vi "Digital Serial Gen Cfg Popup.vi"(8 "error in (no error)":errorcluster, 11 "config file in":path caption="Configuration File") -> (0 "error out":errorcluster, 2 "digital audio protocol settings":T1={"number of channels"=0, "data justification"=enum."Left Justified", "endianness"=enum."LSB First", "channel length"=0, "bit depth"=0, "frame clock rate"=0.0, "bit clock edge sync"=enum."Falling", "master clock rate"=0.0, "Logic Level"=enum."1.2 V", "frame sync edge for channel 0"=enum."Rising", "Channel 0 Offset"=0}, 3 "config file out":path caption="Configuration File")   [LabVIEW 2021, in "Audio Popup UI.lvlib"]
uses:
  Audio Popup UI.lvlib
  controls/digital serial gen settings.ctl
  <vilib>/PDM Acquisition Toolkit/shared/controls/PCM Data Justification.ctl
  <vilib>/PDM Acquisition Toolkit/shared/controls/PCM Bit Endianness.ctl
  <vilib>/PDM Acquisition Toolkit/shared/controls/Digital Edge.ctl
  <vilib>/PDM Acquisition Toolkit/host/Classes/Session/Controls/Logic Levels.ctl
  <vilib>/Utility/miscctls.llb/LVPointTypeDef.ctl
  <vilib>/PDM Acquisition Toolkit/shared/PDM Shared.lvlib
  <vilib>/PDM Acquisition Toolkit/host/Classes/Session/DecoderSession.lvclass
  digital serial gen settings/digital audio protocol controls.lvlib
panel:
  in  "channel 0 offset":u32=1
  in  "Save":bool
  in  "logic level":enum32{"3.3 V", "1.8 V", "1.2 V"}(ring) caption="Logic level"
  in  "master clock rate":dbl=12288000.0 caption="Master clock rate" format="%#_6pHz"
  out "Bit clock rate":dbl=3072000.0 format="%#_6pHz"
  in  "number of channels":u32=2 caption="Number of channels"
  in  "TDM":bool
  in  "RJ":bool
  in  "LJ":bool
  in  "I2S":bool
  in  "bit clock edge sync":enum32{"Rising", "Falling"}(ring)=enum."Falling" caption="Bit clock edge sync"
  in  "frame clock rate":dbl=48000.0 caption="Frame clock rate" format="%#_6pHz"
  in  "data justification":enum32{"Left Justified", "Right Justified"}(ring) caption="Data justification"
  in  "endianness":enum32{"MSB First", "LSB First"}(ring) caption="Endianness"
  in  "bit depth":u32=24 caption="Bit depth"
  in  "channel length":u32=32 caption="Channel length"
  in  "frame sync edge for channel 0":enum32{"Rising", "Falling"}(ring)=enum."Falling" caption="Frame sync edge for Channel 0"
  # "Audio Protocol"
  # "Clock Settings"
  # "Signal Level"
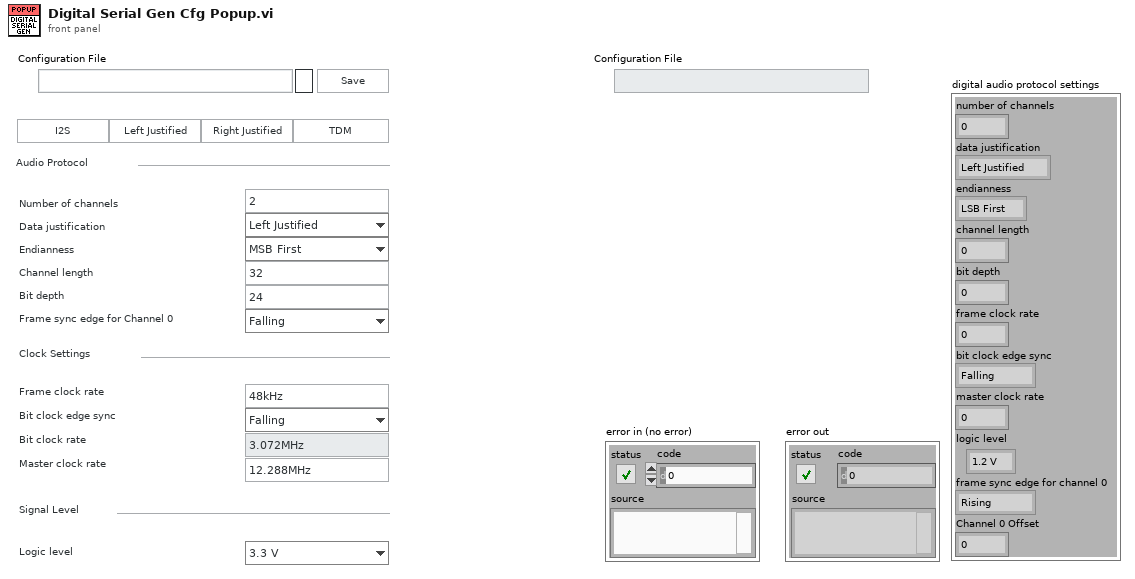
[diagram p1: front panel]
types:
  T1 = typedef "digital serial gen settings.ctl" = cluster{"number of channels":u32, "data justification":T2, "endianness":T3, "channel length":u32, "bit depth":u32, "frame clock rate":dbl, "bit clock edge sync":T4, "master clock rate":dbl, "Logic Level":T5, "frame sync edge for channel 0":T4, "Channel 0 Offset":u32}
  T2 = typedef "PDM Shared.lvlib/PCM Data Justification.ctl" = enum16{"Left Justified", "Right Justified"}
  T3 = typedef "PDM Shared.lvlib/PCM Bit Endianness.ctl" = enum16{"MSB First", "LSB First"}
  T4 = typedef "PDM Shared.lvlib/Digital Edge.ctl" = enum8{"Rising", "Falling"}
  T5 = typedef "PDM Acquisition Class Library.lvlib/DecoderSession.lvclass/Logic Levels.ctl" = enum16{"3.3 V", "1.8 V", "1.2 V"}
  T6 = typedef "LVPointTypeDef.ctl" = cluster{"Horizontal":i16, "Vertical":i16}
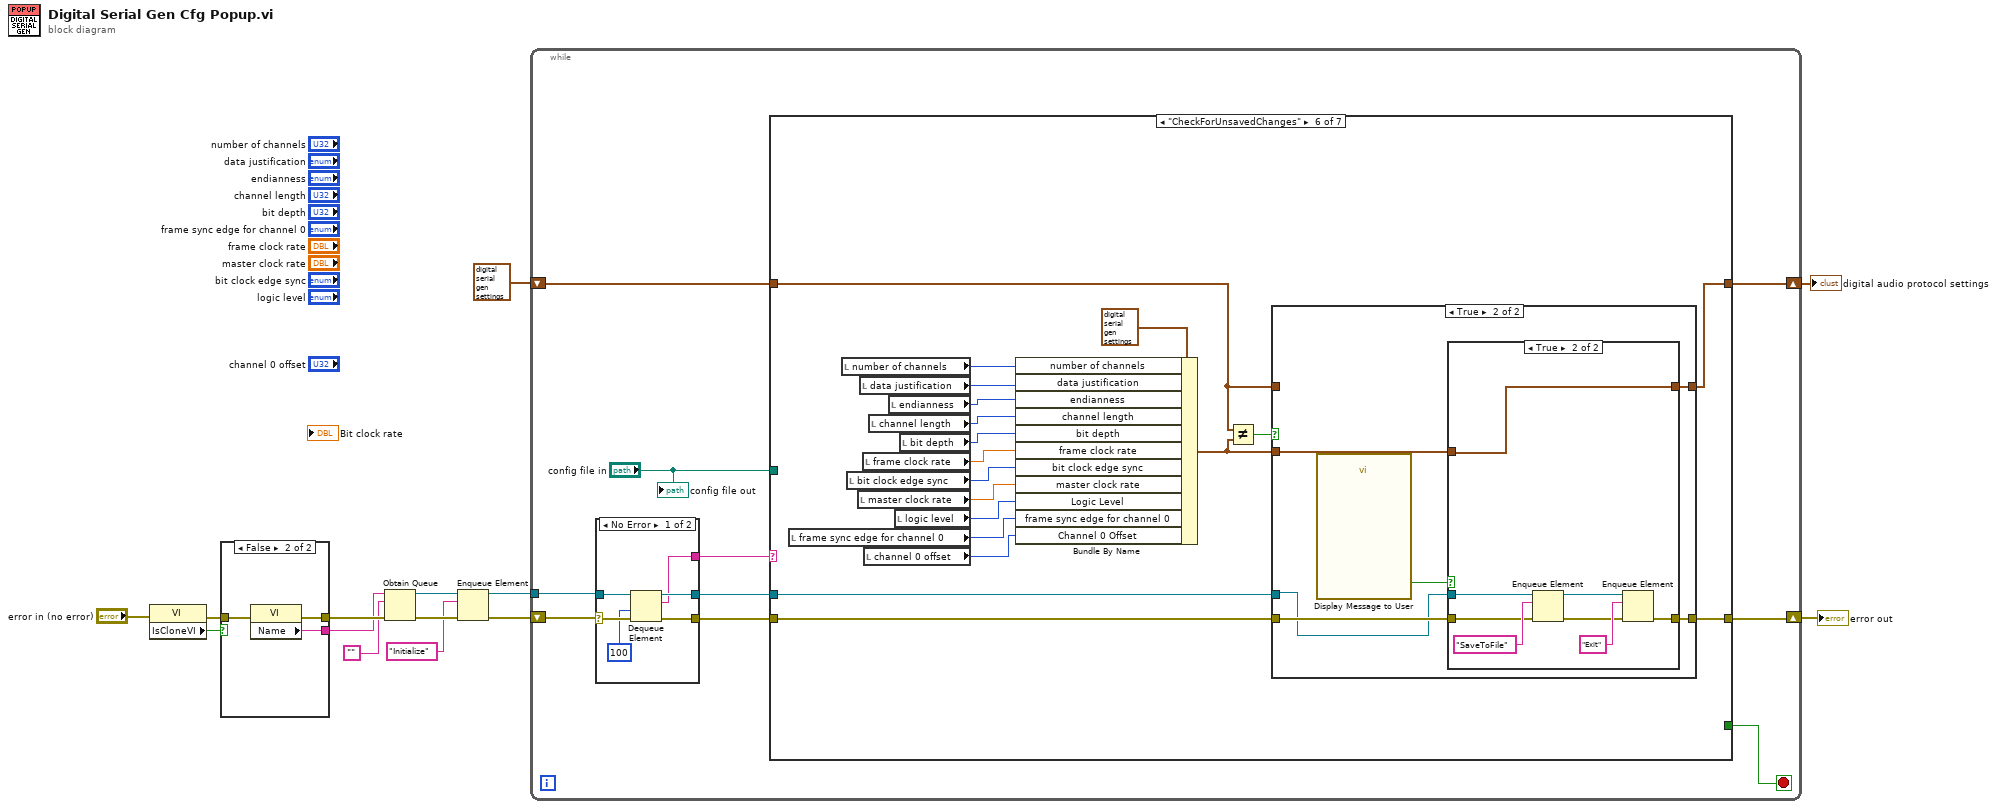
[diagram p0: block diagram]
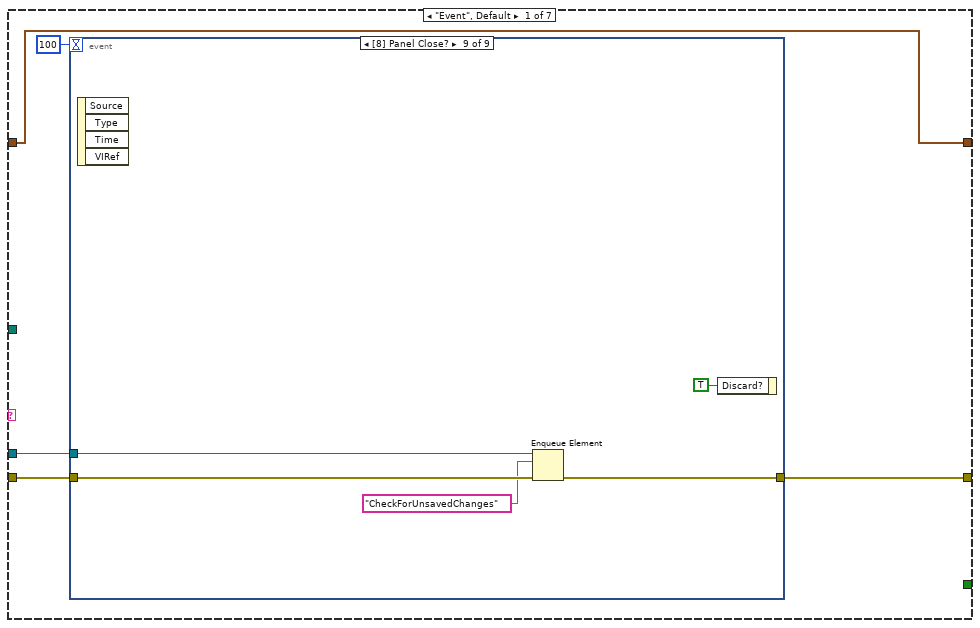
[diagram p2: hidden frame]
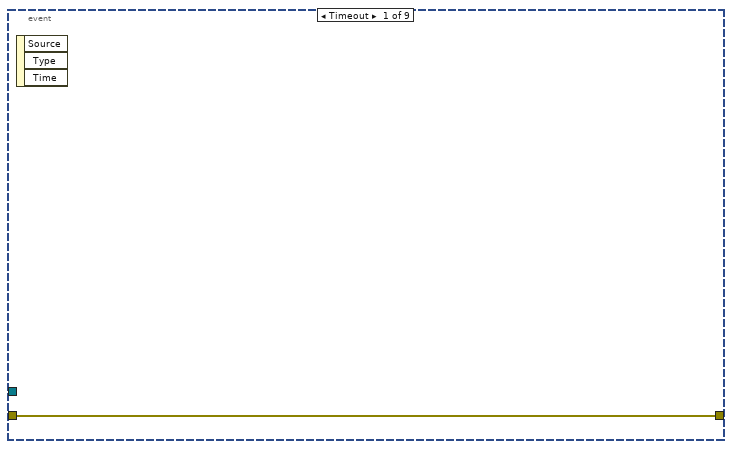
[diagram p3: hidden frame]
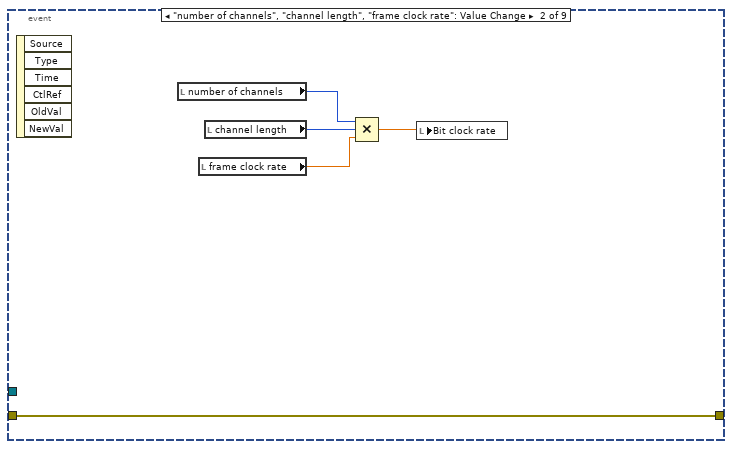
[diagram p4: hidden frame]
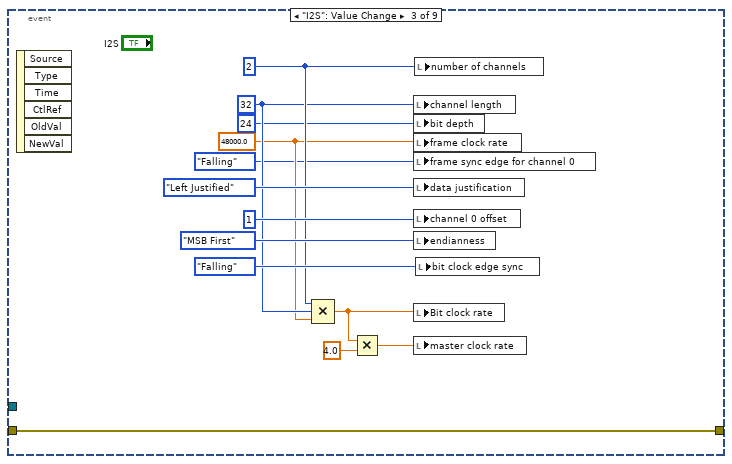
[diagram p5: hidden frame]
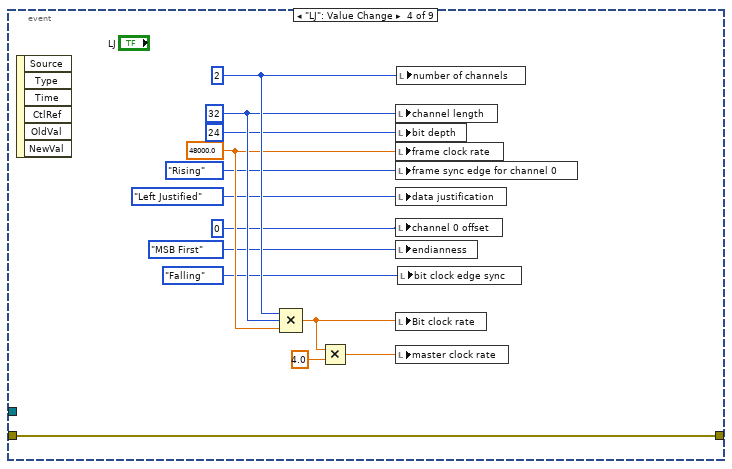
[diagram p6: hidden frame]
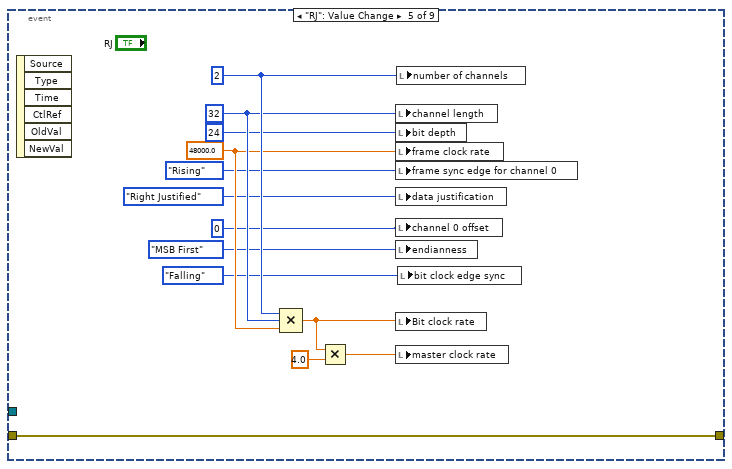
[diagram p7: hidden frame]
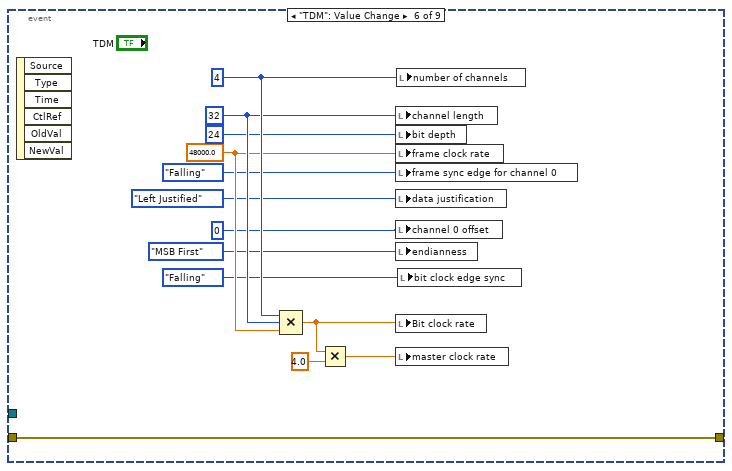
[diagram p8: hidden frame]
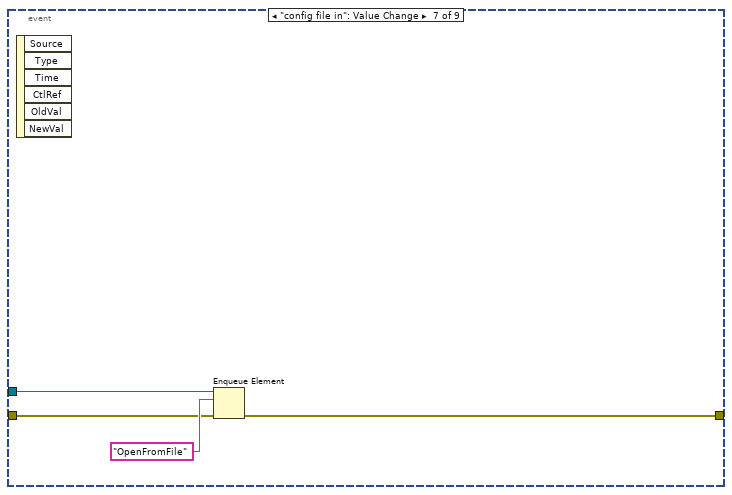
[diagram p9: hidden frame]
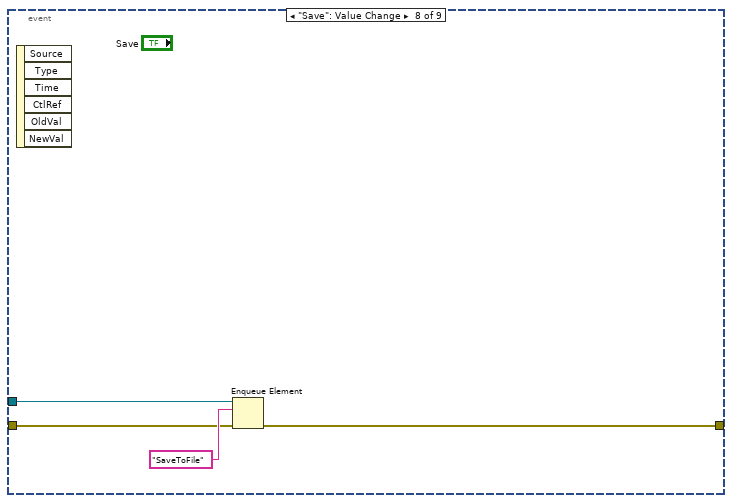
[diagram p10: hidden frame]
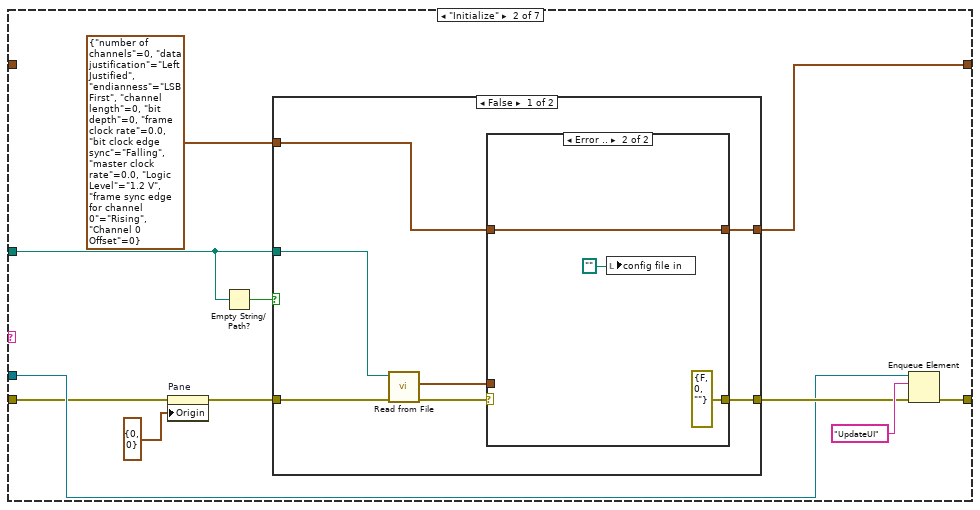
[diagram p11: hidden frame]
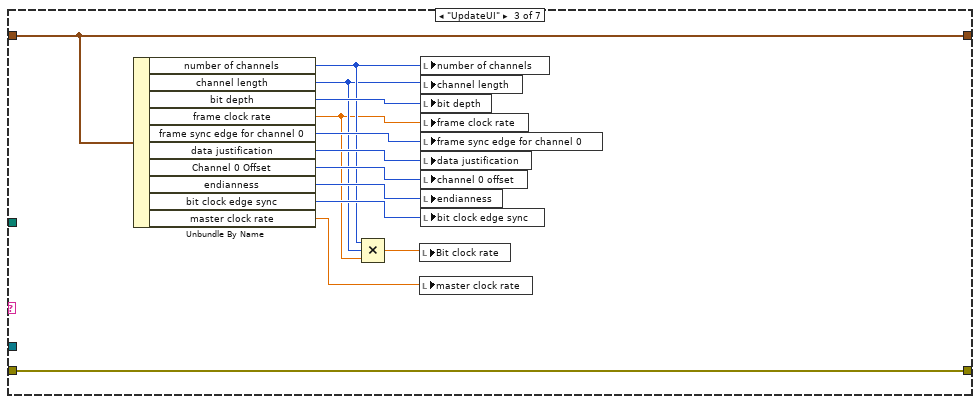
[diagram p14: hidden frame]
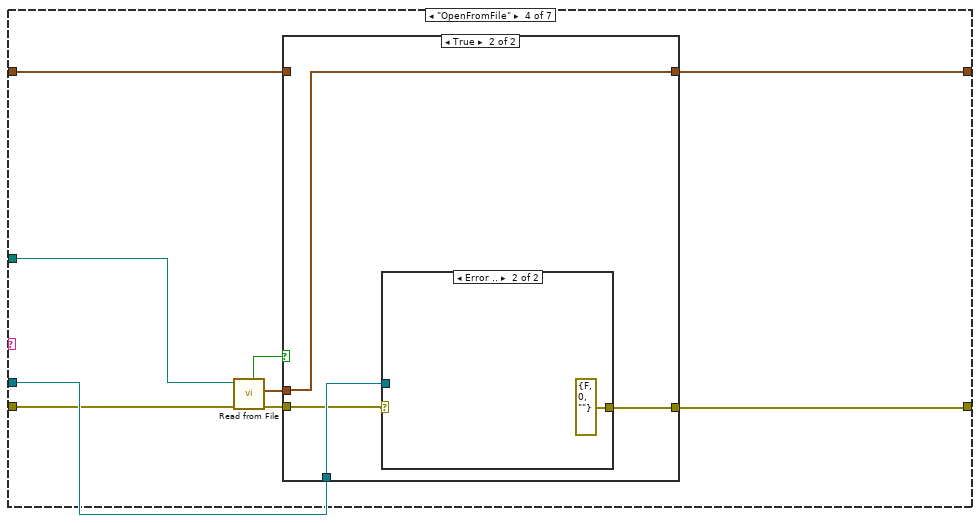
[diagram p15: hidden frame]
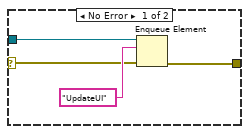
[diagram p17: hidden frame]
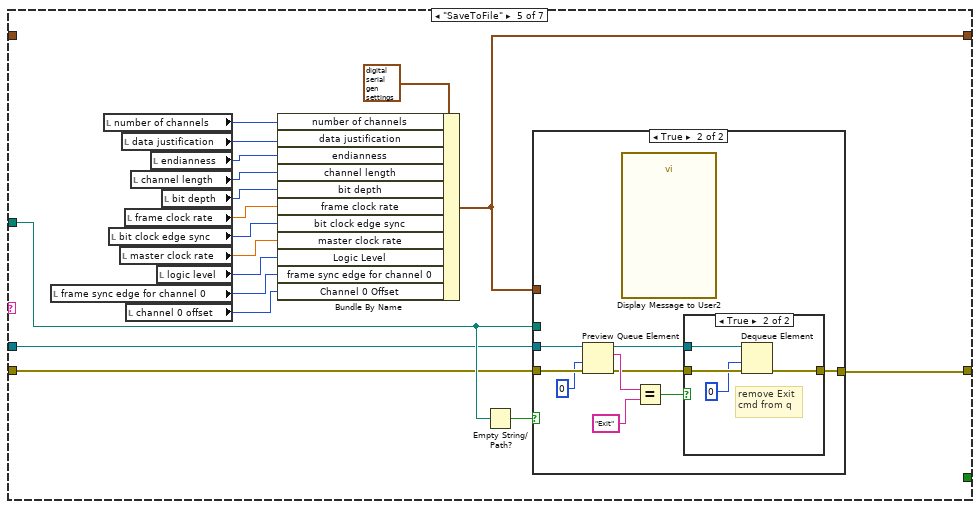
[diagram p18: hidden frame]
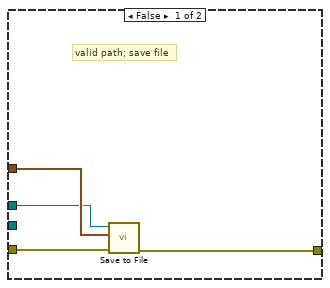
[diagram p19: hidden frame]
diagram:
  n1 = property class="VI"(error in="error in (no error)") -> (error out=w7:errorcluster, "IsCloneVI"=w8:bool)  [unwired: 1 in, 1 out]
  n2 = case shown="False" w8 {
    tunnel: [w17 w20] -> w14
    tunnel: [w16 w19] -> w13
    tunnel: w7 -> [w15 w18]
    frame True {
      n3 = property class="VI"(error in=w15) -> (error out=w17:errorcluster, "Clone Name"=w16:string)  [unwired: 1 in, 1 out]
    }
    frame False {
      n4 = property class="VI"(error in=w18) -> (error out=w20:errorcluster, "Name"=w19:string)  [unwired: 1 in, 1 out]
    }
  }
  n5 = Obtain Queue(name (unnamed)=w13, element data type="", error in (no error)=w14) -> (queue out=w11:refnum<queue>, error out=w12:errorcluster)  [unwired: 2 in, 1 out]
  n6 = Enqueue Element(queue=w11, element="Initialize", error in (no error)=w12) -> (queue out=w5:refnum<queue>, error out=w6:errorcluster)  [unwired: 1 in, 1 out]
  n7 = while {
    tunnel: w5 -> [w29]
    shift-right: [w25] -> w3
    shift-left: w6 -> [w30]
    shift-right: [w22] -> w1
    shift-left: T1 {"number of channels"=0, "data justification"=enum."Left Justified", "endianness"=enum."LSB First", "channel length"=0, "bit depth"=0, "frame clock rate"=0.0, "bit clock edge sync"=enum."Falling", "master clock rate"=0.0, "Logic Level"=enum."1.2 V", "frame sync edge for channel 0"=enum."Rising", "Channel 0 Offset"=0} ("digital audio protocol settings") -> [w23]
    stop <- w24 stop-if-true
    n8 = case shown="No Error" w30 {
      selector: w30 -> [w256 w259]
      tunnel: [w255 w259] -> w26
      tunnel: w29 -> [w254 w258]
      tunnel: [w253 w258] -> w27
      tunnel: [w252 "Handle Error"] -> w28
      frame No Error {
        n9 = Dequeue Element(queue=w254, timeout in ms (-1)=100, error in (no error)=w256) -> (queue out=w253:refnum<queue>, element=w252:string, error out=w255:errorcluster)  [unwired: 1 out]
      }
      frame Error {
      }
    }
    n10 = case shown="\"CheckForUnsavedChanges\"" w28 {
      tunnel: w27 -> [w33 w112 _ w153 w165 w203 w246]
      tunnel: w26 -> [w34 w110 w144 w150 w167 w206 w247]
      tunnel: [w32 w113 w144 w152 w170 w205 w244] -> w25
      tunnel: [_ _ _ _ _ _ TRUE] -> w24
      tunnel: w23 -> [w31 _ w143 w147 _ w201 w243]
      tunnel: [w31 w107 w143 w146 w169 w204 w243] -> w22
      tunnel: "config file in" -> [_ w116 _ w151 w168 _ _]
      frame "Event", Default {
        n11 = event shown="[8] Panel Close?" {
          selector: _ -> [_ _ _ _ _ _ _ _ _]
          dyn-events: _ -> [_ _ _ _ _ _ _ _ _]
          timeout: 100 -> [_ _ _ _ _ _ _ _ _]
          tunnel: w34 -> [w36 w37 w42 w55 w68 w81 w96 w100 w105]
          tunnel: w33 -> [_ _ _ _ _ _ w95 w99 w104]
          tunnel: [w36 w37 w42 w55 w68 w81 w94 w98 w103] -> w32
          event Timeout {
            n12 = event-data() -> ()  [unwired: 1 in, 3 out]
          }
          event "number of channels", "channel length", "frame clock rate": Value Change {
            n13 = event-data() -> ()  [unwired: 1 in, 6 out]
            n14 = local read "number of channels"() -> (w39:u32)
            n15 = local read "frame clock rate"() -> (w38:dbl)
            n16 = local read "channel length"() -> (w40:u32)
            n17 = Compound Arithmetic op=MULTIPLY(w39, w40, w38) -> (w41:dbl)
            n18 = local write "Bit clock rate"(w41) -> ()
          }
          event "I2S": Value Change {
            w45 = 48000.0 ("Frame Clock Rate")
            w46 = u32 32 ("Channel Length")
            w47 = u32 2 ("Number of Channels")
            n19 = event-data() -> ()  [unwired: 1 in, 6 out]
            n20 = Compound Arithmetic op=MULTIPLY(w47, w46, w45) -> (w53:dbl)
            n21 = Multiply(x=w53, y=4.0) -> (x*y=w52:dbl)
            n22 = local write "channel length"(w46) -> ()
            n23 = local write "bit depth"(u32 24 ("Bit Depth")) -> ()
            n24 = local write "frame clock rate"(w45) -> ()
            n25 = local write "frame sync edge for channel 0"(enum32{"Rising", "Falling"}."Falling" ("bit clock edge sync")) -> ()
            n26 = local write "data justification"(enum32{"Left Justified", "Right Justified"}."Left Justified" ("data justification")) -> ()
            n27 = local write "channel 0 offset"(u32 1 ("Channel 0 Offset")) -> ()
            n28 = local write "endianness"(enum32{"MSB First", "LSB First"}."MSB First" ("endianness")) -> ()
            n29 = local write "Bit clock rate"(w53) -> ()
            n30 = local write "master clock rate"(w52) -> ()
            n31 = local write "number of channels"(w47) -> ()
            n32 = local write "bit clock edge sync"(enum32{"Rising", "Falling"}."Falling" ("frame sync edge for channel 0")) -> ()
          }
          event "LJ": Value Change {
            w63 = 48000.0 ("Frame Clock Rate")
            w65 = u32 32 ("Channel Length")
            w66 = u32 2 ("Number of Channels")
            n33 = event-data() -> ()  [unwired: 1 in, 6 out]
            n34 = Compound Arithmetic op=MULTIPLY(w66, w65, w63) -> (w57:dbl)
            n35 = Multiply(x=w57, y=4.0) -> (x*y=w56:dbl)
            n36 = local write "channel length"(w65) -> ()
            n37 = local write "bit depth"(u32 24 ("Bit Depth")) -> ()
            n38 = local write "frame clock rate"(w63) -> ()
            n39 = local write "frame sync edge for channel 0"(enum32{"Rising", "Falling"}."Rising" ("bit clock edge sync")) -> ()
            n40 = local write "data justification"(enum32{"Left Justified", "Right Justified"}."Left Justified" ("data justification")) -> ()
            n41 = local write "channel 0 offset"(u32 0 ("Channel 0 Offset")) -> ()
            n42 = local write "endianness"(enum32{"MSB First", "LSB First"}."MSB First" ("endianness")) -> ()
            n43 = local write "Bit clock rate"(w57) -> ()
            n44 = local write "master clock rate"(w56) -> ()
            n45 = local write "number of channels"(w66) -> ()
            n46 = local write "bit clock edge sync"(enum32{"Rising", "Falling"}."Falling" ("frame sync edge for channel 0")) -> ()
          }
          event "RJ": Value Change {
            w76 = 48000.0 ("Frame Clock Rate")
            w78 = u32 32 ("Channel Length")
            w79 = u32 2 ("Number of Channels")
            n47 = event-data() -> ()  [unwired: 1 in, 6 out]
            n48 = Compound Arithmetic op=MULTIPLY(w79, w78, w76) -> (w70:dbl)
            n49 = Multiply(x=w70, y=4.0) -> (x*y=w69:dbl)
            n50 = local write "channel length"(w78) -> ()
            n51 = local write "bit depth"(u32 24 ("Bit Depth")) -> ()
            n52 = local write "frame clock rate"(w76) -> ()
            n53 = local write "frame sync edge for channel 0"(enum32{"Rising", "Falling"}."Rising" ("bit clock edge sync")) -> ()
            n54 = local write "data justification"(enum32{"Left Justified", "Right Justified"}."Right Justified" ("data justification")) -> ()
            n55 = local write "channel 0 offset"(u32 0 ("Channel 0 Offset")) -> ()
            n56 = local write "endianness"(enum32{"MSB First", "LSB First"}."MSB First" ("endianness")) -> ()
            n57 = local write "Bit clock rate"(w70) -> ()
            n58 = local write "master clock rate"(w69) -> ()
            n59 = local write "number of channels"(w79) -> ()
            n60 = local write "bit clock edge sync"(enum32{"Rising", "Falling"}."Falling" ("frame sync edge for channel 0")) -> ()
          }
          event "TDM": Value Change {
            w89 = 48000.0 ("Frame Clock Rate")
            w91 = u32 32 ("Channel Length")
            w92 = u32 4 ("Number of Channels")
            n61 = event-data() -> ()  [unwired: 1 in, 6 out]
            n62 = Compound Arithmetic op=MULTIPLY(w92, w91, w89) -> (w83:dbl)
            n63 = Multiply(x=w83, y=4.0) -> (x*y=w82:dbl)
            n64 = local write "channel length"(w91) -> ()
            n65 = local write "bit depth"(u32 24 ("Bit Depth")) -> ()
            n66 = local write "frame clock rate"(w89) -> ()
            n67 = local write "frame sync edge for channel 0"(enum32{"Rising", "Falling"}."Falling" ("bit clock edge sync")) -> ()
            n68 = local write "data justification"(enum32{"Left Justified", "Right Justified"}."Left Justified" ("data justification")) -> ()
            n69 = local write "channel 0 offset"(u32 0 ("Channel 0 Offset")) -> ()
            n70 = local write "endianness"(enum32{"MSB First", "LSB First"}."MSB First" ("endianness")) -> ()
            n71 = local write "Bit clock rate"(w83) -> ()
            n72 = local write "master clock rate"(w82) -> ()
            n73 = local write "number of channels"(w92) -> ()
            n74 = local write "bit clock edge sync"(enum32{"Rising", "Falling"}."Falling" ("frame sync edge for channel 0")) -> ()
          }
          event "config file in": Value Change {
            n75 = event-data() -> ()  [unwired: 1 in, 6 out]
            n76 = Enqueue Element(queue=w95, element="OpenFromFile", error in (no error)=w96) -> (error out=w94:errorcluster)  [unwired: 1 in, 2 out]
          }
          event "Save": Value Change {
            n77 = event-data() -> ()  [unwired: 1 in, 6 out]
            n78 = Enqueue Element(queue=w99, element="SaveToFile", error in (no error)=w100) -> (error out=w98:errorcluster)  [unwired: 1 in, 2 out]
          }
          event Panel Close? {
            n79 = event-data() -> ()  [unwired: 1 in, 4 out]
            n80 = Enqueue Element(queue=w104, element="CheckForUnsavedChanges", error in (no error)=w105) -> (error out=w103:errorcluster)  [unwired: 1 in, 2 out]
            n81 = event-data("Discard?"=TRUE) -> ()  [unwired: 1 in, 1 out]
          }
        }
      }
      frame "Initialize" {
        n82 = property on="Pane" class="Pane"(error in=w110, "Origin"=T6 {"Horizontal"=0, "Vertical"=0}) -> (error out=w109:errorcluster)  [unwired: 1 in, 1 out]
        n83 = Empty String/Path?(string/path=w116) -> (empty?=w117:bool)
        n84 = case shown="False" w117 {
          tunnel: w109 -> [w124 w131]
          tunnel: w116 -> [w123 _]
          tunnel: [w119 w130] -> w107
          tunnel: [w121 w131] -> w114
          tunnel: T1 {"number of channels"=0, "data justification"=enum."Left Justified", "endianness"=enum."LSB First", "channel length"=0, "bit depth"=0, "frame clock rate"=0.0, "bit clock edge sync"=enum."Falling", "master clock rate"=0.0, "Logic Level"=enum."1.2 V", "frame sync edge for channel 0"=enum."Rising", "Channel 0 Offset"=0} ("digital audio protocol settings") -> [w118 w130]
          frame False {
            n85 = call "Read from File.vi"("error in (no error)"=w124, "file path"=w123) -> ("error out"=w122:errorcluster, "digital audio protocol settings"=w120:T1)  [unwired: 7 in, 1 out]
            n86 = case shown="Error .." w122 {
              selector: w122 -> [w126 _]
              tunnel: [w126 errorcluster {"status"=FALSE, "code"=0, "source"=""} ("error IO")] -> w121
              tunnel: w120 -> [w125 _]
              tunnel: [w125 w129] -> w119
              tunnel: w118 -> [_ w129]
              frame No Error {
              }
              frame Error {
                n87 = local write "config file in"(path "") -> ()
              }
            }
          }
          frame True {
          }
        }
        n88 = Enqueue Element(queue=w112, element="UpdateUI", error in (no error)=w114) -> (error out=w113:errorcluster)  [unwired: 1 in, 2 out]
      }
      frame "UpdateUI" {
        n89 = Unbundle By Name(w143) -> ("number of channels"=w136:u32, "channel length"=w135:u32, "bit depth"=w142:u32, "frame clock rate"=w134:dbl, "frame sync edge for channel 0"=w141:T4, "data justification"=w140:T2, "Channel 0 Offset"=w139:u32, "endianness"=w138:T3, "bit clock edge sync"=w137:T4, "master clock rate"=w132:dbl)
        n90 = Compound Arithmetic op=MULTIPLY(w136, w135, w134) -> (w133:dbl)
        n91 = local write "Bit clock rate"(w133) -> ()
        n92 = local write "master clock rate"(w132) -> ()
        n93 = local write "number of channels"(w136) -> ()
        n94 = local write "channel length"(w135) -> ()
        n95 = local write "bit depth"(w142) -> ()
        n96 = local write "frame clock rate"(w134) -> ()
        n97 = local write "frame sync edge for channel 0"(w141) -> ()
        n98 = local write "data justification"(w140) -> ()
        n99 = local write "channel 0 offset"(w139) -> ()
        n100 = local write "endianness"(w138) -> ()
        n101 = local write "bit clock edge sync"(w137) -> ()
      }
      frame "OpenFromFile" {
        n102 = call "Read from File.vi"("error in (no error)"=w150, "file path"=w151) -> ("error out"=w149:errorcluster, "digital audio protocol settings"=w145:T1, "file exists?"=w148:bool)  [unwired: 7 in]
        n103 = case shown="True" w148 {
          tunnel: w153 -> [_ w159]
          tunnel: [w154 w158] -> w152
          tunnel: w149 -> [w154 w156]
          tunnel: w147 -> [w155 _]
          tunnel: [w155 w157] -> w146
          tunnel: w145 -> [_ w157]
          frame False {
          }
          frame True {
            n104 = case shown="Error .." w156 {
              selector: w156 -> [w160 _]
              tunnel: w159 -> [w162 _]
              tunnel: [w161 errorcluster {"status"=FALSE, "code"=0, "source"=""} ("error out")] -> w158
              frame No Error {
                n105 = Enqueue Element(queue=w162, element="UpdateUI", error in (no error)=w160) -> (error out=w161:errorcluster)  [unwired: 1 in, 2 out]
              }
              frame Error {
              }
            }
          }
        }
      }
      frame "SaveToFile" {
        n106 = local read "frame sync edge for channel 0"() -> (w172:enum32{"Rising", "Falling"})
        n107 = local read "number of channels"() -> (w181:u32)
        n108 = local read "bit clock edge sync"() -> (w175:enum32{"Rising", "Falling"})
        n109 = local read "master clock rate"() -> (w174:dbl)
        n110 = local read "data justification"() -> (w180:enum32{"Left Justified", "Right Justified"})
        n111 = local read "frame clock rate"() -> (w176:dbl)
        n112 = local read "channel 0 offset"() -> (w171:u32)
        n113 = local read "channel length"() -> (w178:u32)
        n114 = local read "endianness"() -> (w179:enum32{"MSB First", "LSB First"})
        n115 = local read "logic level"() -> (w173:enum32{"3.3 V", "1.8 V", "1.2 V"})
        n116 = local read "bit depth"() -> (w177:u32)
        n117 = Bundle By Name(cluster=T1 {"number of channels"=0, "data justification"=enum."Left Justified", "endianness"=enum."LSB First", "channel length"=0, "bit depth"=0, "frame clock rate"=0.0, "bit clock edge sync"=enum."Falling", "master clock rate"=0.0, "Logic Level"=enum."1.2 V", "frame sync edge for channel 0"=enum."Rising", "Channel 0 Offset"=0} ("input cluster"), "number of channels"=w181, "data justification"=w180, "endianness"=w179, "channel length"=w178, "bit depth"=w177, "frame clock rate"=w176, "bit clock edge sync"=w175, "master clock rate"=w174, "Logic Level"=w173, "frame sync edge for channel 0"=w172, "Channel 0 Offset"=w171) -> (w169:T1)
        n118 = Empty String/Path?(string/path=w168) -> (empty?=w166:bool)
        n119 = case shown="True" w166 {
          tunnel: [w186 w188] -> w170
          tunnel: w169 -> [w185 _]
          tunnel: w168 -> [w184 _]
          tunnel: w167 -> [w183 w195]
          tunnel: w165 -> [_ w194]
          frame False {
            # "valid path; save file"
            n120 = call "Save to File.vi"("error in (no error)"=w183, "digital audio protocol settings"=w185, "file path"=w184) -> ("error out"=w186:errorcluster)  [unwired: 8 in]
          }
          frame True {
            n121 = Preview Queue Element(queue=w194, timeout in ms (-1)=0, error in (no error)=w195) -> (queue out=w191:refnum<queue>, element=w193:string, error out=w189:errorcluster)  [unwired: 1 out]
            n122 = call "Display Message to User2"() -> ()  [unwired: 10 in, 2 out]
            n123 = Equal?(x=w193, y="Exit") -> (x = y?=w190:bool)
            n124 = case shown="True" w190 {
              tunnel: w191 -> [_ w200]
              tunnel: w189 -> [w196 w199]
              tunnel: [w196 w198] -> w188
              frame False {
              }
              frame True {
                # "remove Exit\ncmd from q"
                n125 = Dequeue Element(queue=w200, timeout in ms (-1)=0, error in (no error)=w199) -> (error out=w198:errorcluster)  [unwired: 3 out]
              }
            }
          }
        }
      }
      frame "CheckForUnsavedChanges" {
        n126 = local read "frame sync edge for channel 0"() -> (w210:enum32{"Rising", "Falling"})
        n127 = local read "number of channels"() -> (w219:u32)
        n128 = local read "bit clock edge sync"() -> (w213:enum32{"Rising", "Falling"})
        n129 = local read "master clock rate"() -> (w212:dbl)
        n130 = local read "data justification"() -> (w218:enum32{"Left Justified", "Right Justified"})
        n131 = local read "frame clock rate"() -> (w214:dbl)
        n132 = local read "channel 0 offset"() -> (w209:u32)
        n133 = local read "channel length"() -> (w216:u32)
        n134 = local read "endianness"() -> (w217:enum32{"MSB First", "LSB First"})
        n135 = local read "logic level"() -> (w211:enum32{"3.3 V", "1.8 V", "1.2 V"})
        n136 = local read "bit depth"() -> (w215:u32)
        n137 = Bundle By Name(cluster=T1 {"number of channels"=0, "data justification"=enum."Left Justified", "endianness"=enum."LSB First", "channel length"=0, "bit depth"=0, "frame clock rate"=0.0, "bit clock edge sync"=enum."Falling", "master clock rate"=0.0, "Logic Level"=enum."1.2 V", "frame sync edge for channel 0"=enum."Rising", "Channel 0 Offset"=0} ("input cluster"), "number of channels"=w219, "data justification"=w218, "endianness"=w217, "channel length"=w216, "bit depth"=w215, "frame clock rate"=w214, "bit clock edge sync"=w213, "master clock rate"=w212, "Logic Level"=w211, "frame sync edge for channel 0"=w210, "Channel 0 Offset"=w209) -> (w202:T1)
        n138 = Not Equal?(x=w201, y=w202) -> (x != y?=w207:bool)
        n139 = case shown="True" w207 {
          tunnel: w206 -> [w222 w230]
          tunnel: [w220 w226] -> w205
          tunnel: w202 -> [_ w228]
          tunnel: w201 -> [w224 _]
          tunnel: [w224 w227] -> w204
          tunnel: w203 -> [w221 w225]
          frame False {
            n140 = Enqueue Element(queue=w221, element="Exit", error in (no error)=w222) -> (error out=w220:errorcluster)  [unwired: 1 in, 2 out]
          }
          frame True {
            n141 = call "Display Message to User"() -> ("Yes"=w229:bool)  [unwired: 10 in, 1 out]
            n142 = case shown="True" w229 {
              tunnel: w230 -> [w234 w241]
              tunnel: w228 -> [_ w240]
              tunnel: [_ w240] -> w227
              tunnel: [w232 w236] -> w226
              tunnel: w225 -> [w233 w235]
              frame False {
                n143 = Enqueue Element(queue=w233, element="Exit", error in (no error)=w234) -> (error out=w232:errorcluster)  [unwired: 1 in, 2 out]
              }
              frame True {
                n144 = Enqueue Element(queue=w235, element="SaveToFile", error in (no error)=w241) -> (queue out=w237:refnum<queue>, error out=w238:errorcluster)  [unwired: 1 in, 1 out]
                n145 = Enqueue Element(queue=w237, element="Exit", error in (no error)=w238) -> (error out=w236:errorcluster)  [unwired: 1 in, 2 out]
              }
            }
          }
        }
      }
      frame "Exit" {
        n146 = Flush Queue(queue=w246, error in (no error)=w247) -> (queue out=w250:refnum<queue>, error out=w249:errorcluster)  [unwired: 1 out]
        n147 = Release Queue(queue=w250, force destroy? (F)=TRUE, error in (no error)=w249) -> (error out=w244:errorcluster)  [unwired: 2 out]
      }
    }
    "config file out" <- "config file in"
  }
  "error out" <- w3
  "digital audio protocol settings" <- w1
